vi "SENS_SWE_TYPE.vi"(0 "VISA IN":refnum<visa-resource-name>, 1 "Sweep Type":string(combo)="LINear", 5 "error in":errorcluster, 7 "Channel":i32=1) -> (14 "VISA Out":refnum<visa-resource-name>, 19 "error out":errorcluster)   [LabVIEW 2018, in "PNA-X.lvlib"]
doc: "SENSe<cnum>:SWEep:TYPE <char> \n1820\n\n(Read-Write) Sets the type of analyzer sweep mode. \nParameters \n<cnum> Any existing channel number. If unspecified, value is set to 1 \n<char> Choose from: \nLINear | LOGarithmic | POWer | CW | SEGMent \nNote: SWEep TYPE cannot be set to SEGMent if there are no segments turned ON. A \nsegment is automatically turned ON when the analyzer is started. \nExamples SENS:SWE:TYPE LIN \nsense2:sweep:type segment \nQuery Syntax SENSe<cnum>:SWEep:TYPE? \nReturn Type Character \nDefault LINear \nLast Modified: \n24-Apr-2007 Clarified Sweep mode \n1821\n\nX Values Command"
uses:
  PNA-X.lvlib
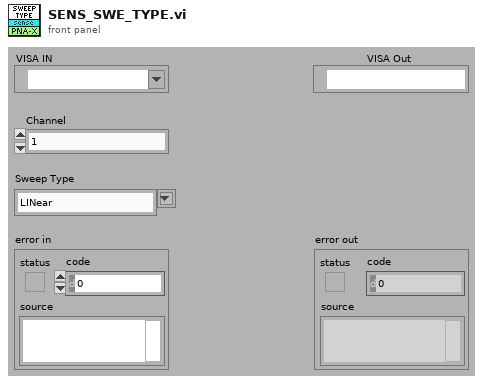
[diagram p1: front panel]
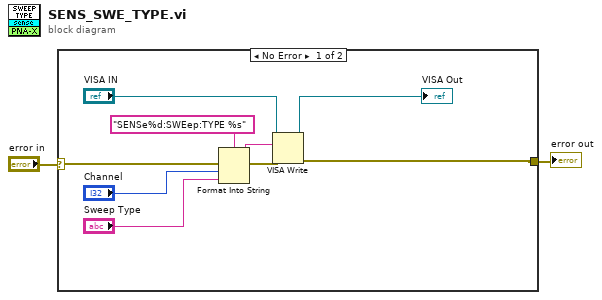
[diagram p0: block diagram]
diagram:
  n1 = case shown="No Error" "error in" {
    selector: "error in" -> [w11 w12]
    tunnel: [w6 w12] -> w1
    frame No Error {
      n2 = Format Into String(format string="SENSe%d:SWEep:TYPE %s" ("Cmdline"), error in=w11, "Channel", "Sweep Type") -> (resulting string=w9:string, error out=w10:errorcluster)  [unwired: 1 in]
      n3 = VISA Write(VISA resource name="VISA IN", write buffer=w9, error in (no error)=w10) -> (VISA resource name out=→"VISA Out":refnum<visa-resource-name>, error out=w6:errorcluster)  [unwired: 1 out]
    }
    frame Error {
    }
  }
  "error out" <- w1
